vi "Instructor Log.vi"() -> ()   [LabVIEW 2017]
uses:
  <vilib>/OPCUA/controls/Write Status.ctl
  <vilib>/OPCUA/controls/NodeId.ctl
  <vilib>/OPCUA/client/Multiple Write String.vi
  <vilib>/OPCUA/NI OPC UA Client.lvlib
panel:
  out "Log Loop":i32
  out "Send Loop":i32
  in  "Stop Log":bool
  out "Chat Window":string
  in  "Node Status":T1 items=["Good"=0, "Uncertain_InitialValue"=1083310080, "Uncertain_LastUsableValue"=1083179008, "Uncertain_SensorNotAccurate"=1083375616, "Uncertain_EngineeringUnitsExceeded"=1083441152, "Bad_NoCommunication"=2150694912, "Bad_NotReadable"=2151284736, "Bad_NotWritable"=2151350272, "Bad_OutOfRange"=2151415808, "Bad_WaitingForInitialData"=2150760448]
  in  "Time Stamp":timestamp
  in  "Enter Text":string
  in  "Node Status":T1 items=["Good"=0, "Uncertain_InitialValue"=1083310080, "Uncertain_LastUsableValue"=1083179008, "Uncertain_SensorNotAccurate"=1083375616, "Uncertain_EngineeringUnitsExceeded"=1083441152, "Bad_NoCommunication"=2150694912, "Bad_NotReadable"=2151284736, "Bad_NotWritable"=2151350272, "Bad_OutOfRange"=2151415808, "Bad_WaitingForInitialData"=2150760448]
  in  "Time Stamp":timestamp
  in  "Stop Chat":bool
  in  "Send":bool
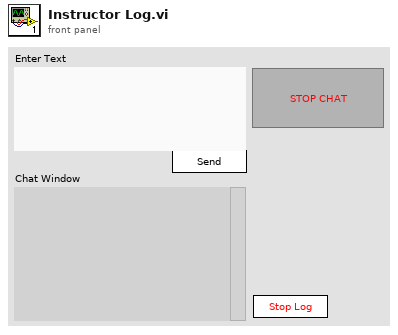
[diagram p1: front panel]
types:
  T1 = typedef "Write Status.ctl" = u32
  T2 = cluster{"message mode":enum16{"None", "Sign", "Sign and Encrypt"}, "security":enum16{"Basic256", "Basic128Rsa15"}}
  T3 = enum16{"open", "replace", "create", "open or create", "replace or create", "replace or create with confirmation"}
  T4 = typedef "OPC UA Client Refnum.ctl" = refnum<k21>
  T5 = typedef "NodeId.ctl" = string
  T6 = cluster{"node ID":T5, "value":string, "timestamp (current time)":timestamp, "node status":T1}
  T7 = cluster{"node ID":T5, "value":string, "timestamp (current time)":timestamp, "node status":T1}[]
  T8 = typedef "Subscription ID.ctl" = u32
  T9 = typedef "Subscription Data Change.ctl" = cluster{"node ID":T5, " value":variant, "timestamp":timestamp, "data type":T10, "status code":T11}
  T10 = typedef "Data Type.ctl" = u16
  T11 = typedef "OPC UA StatusCode.ctl" = u32
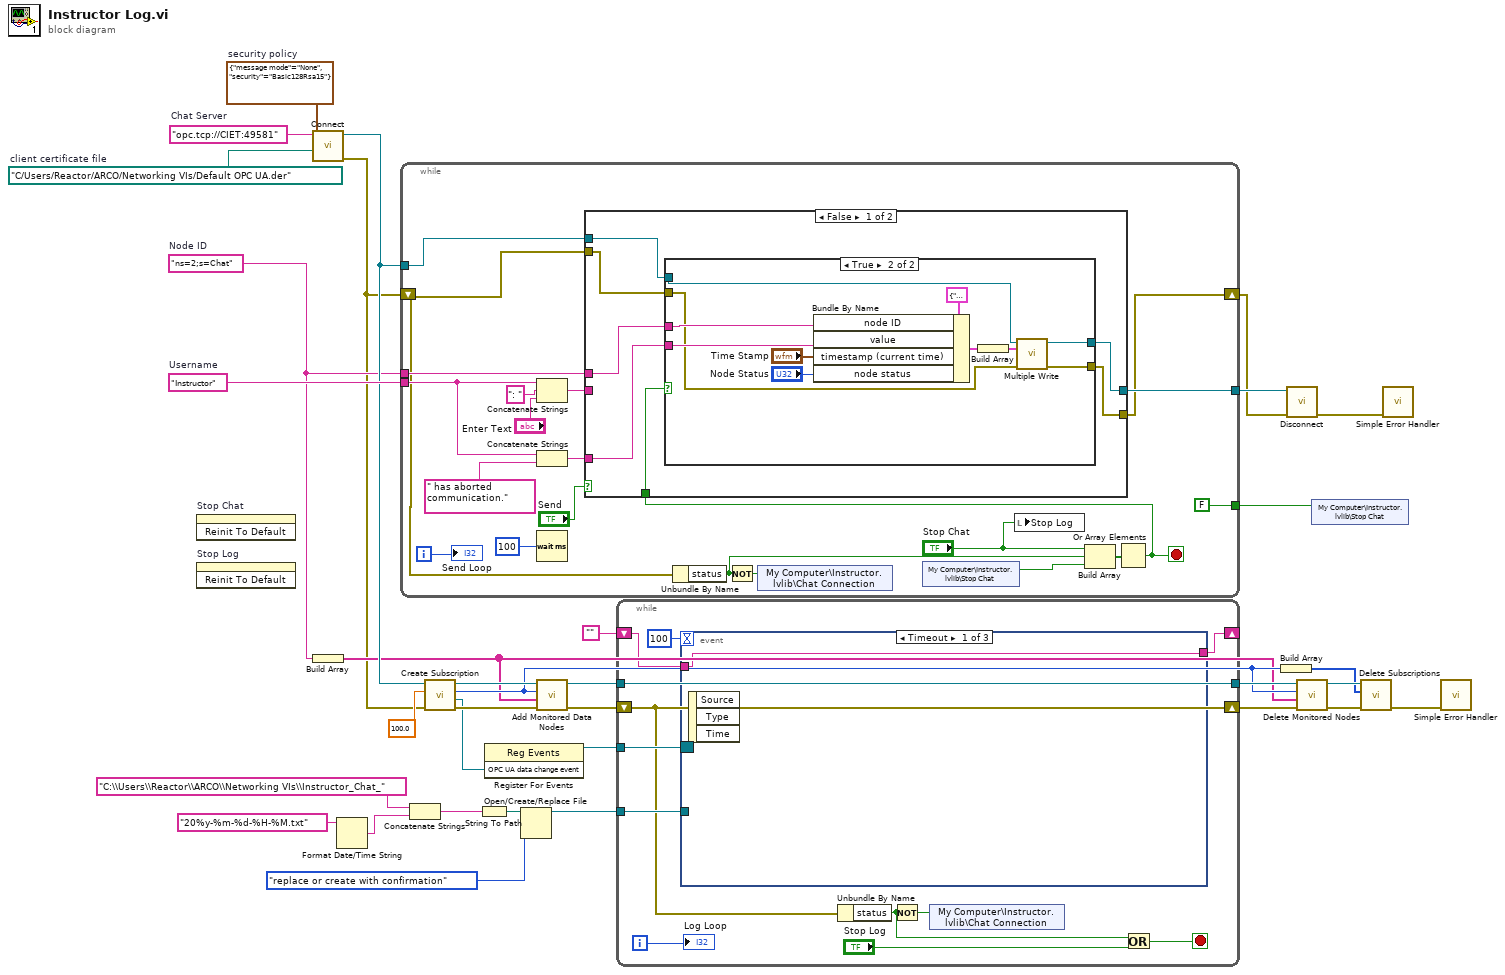
[diagram p0: block diagram]
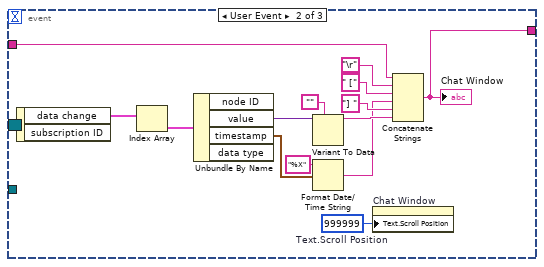
[diagram p2: hidden frame]
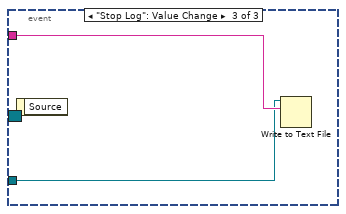
[diagram p3: hidden frame]
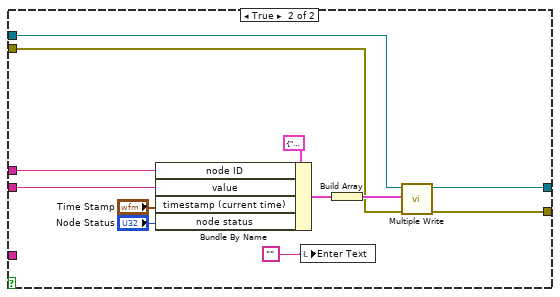
[diagram p5: hidden frame]
diagram:
  w12 = T2 {"message mode"=enum."None", "security"=enum."Basic128Rsa15"}  # security policy
  w13 = path "C:/Users/Reactor/ARCO/Networking VIs/Default OPC UA.der"  # client certificate file
  w17 = "ns=2;s=Chat"  # Node ID
  w32 = "Instructor"  # Username
  w33 = "opc.tcp://CIET:49581"  # Chat Server
  n1 = invoke on="Stop Chat" class="Bool (strict)" method="Reinit To Default"() -> ()  [unwired: 3 in, 3 out]
  n2 = invoke on="Stop Log" class="Bool (strict)" method="Reinit To Default"() -> ()  [unwired: 3 in, 3 out]
  n3 = call <vilib>:"Connect.vi"("client certificate file"=w13, "security policy"=w12, "server endpoint URL"=w33) -> ("error out"=w9:errorcluster, "OPC UA client refnum out"=w31:T4)  [unwired: 6 in, 1 out]
  n4 = Build Array(w17) -> (w16:string[])
  n5 = Format Date/Time String(time format string (%c)="20%y-%m-%d-%H-%M.txt") -> (date/time string=w4:string)  [unwired: 2 in]
  n6 = while {
    tunnel: w17 -> [w47]
    tunnel: w32 -> [w52]
    tunnel: w31 -> [w45]
    tunnel: [w46] -> w14
    tunnel: [FALSE] -> w10
    shift-right: [w36] -> w7
    shift-left: w9 -> [w35]
    i -> [w50]
    stop <- w41 stop-if-true
    n7 = Concatenate Strings(w52, ": ", "Enter Text") -> (w48:string)
    n8 = Concatenate Strings(w52, " has aborted communication.") -> (w44:string)
    n9 = Wait (ms)(milliseconds to wait=u32 100) -> ()  [unwired: 1 out]
    n10 = Unbundle By Name(w35) -> ("status"=w39:bool)
    n11 = Not(x=w39) -> (.not. x?=w42:bool)
    n12 = shared-variable "My Computer\\Instructor.lvlib\\Chat Connection"(w42) -> ()  [unwired: 1 in, 1 out]
    n13 = shared-variable "My Computer\\Instructor.lvlib\\Stop Chat"() -> (w40:bool)  [unwired: 1 in, 1 out]
    n14 = local write "Stop Log"("Stop Chat") -> ()
    n15 = Build Array("Stop Chat", w39, w40) -> (w37:bool[])
    n16 = Or Array Elements(Boolean array=w37) -> (logical OR=w41:bool)
    n17 = case shown="False" "Send" {
      tunnel: w48 -> [_ w82]
      tunnel: w47 -> [w60 w81]
      tunnel: [w56 w79] -> w46
      tunnel: [w57 w78] -> w36
      tunnel: w45 -> [w58 w77]
      tunnel: w35 -> [w59 w76]
      tunnel: w41 -> [w62 _]
      tunnel: w44 -> [w61 _]
      frame False {
        n18 = case shown="True" w62 {
          tunnel: w61 -> [_ w70]
          tunnel: w60 -> [_ w69]
          tunnel: w59 -> [w63 w68]
          tunnel: w58 -> [w64 w67]
          tunnel: [w64 w66] -> w56
          tunnel: [w63 w65] -> w57
          frame False {
          }
          frame True {
            n19 = Bundle By Name(cluster=T6 {"node ID"="", "value"="", "timestamp (current time)"=timestamp(0 s since 1904-01-01), "node status"=0} ("request"), "node ID"=w69, "value"=w70, "timestamp (current time)"="Time Stamp", "node status"="Node Status") -> (w73:T6)
            n20 = Build Array(w73) -> (w72:T7)
            n21 = call-poly <vilib>:"Multiple Write.vi"("error in (no error)"=w68, "requests"=w72, "OPC UA client refnum in"=w67) -> ("error out"=w65:errorcluster, "OPC UA client refnum out"=w66:T4)  [unwired: 5 in, 2 out]
          }
        }
      }
      frame True {
        n22 = Bundle By Name(cluster=T6 {"node ID"="", "value"="", "timestamp (current time)"=timestamp(0 s since 1904-01-01), "node status"=0} ("request"), "node ID"=w81, "value"=w82, "timestamp (current time)"="Time Stamp", "node status"="Node Status") -> (w85:T6)
        n23 = local write "Enter Text"("") -> ()
        n24 = Build Array(w85) -> (w84:T7)
        n25 = call-poly <vilib>:"Multiple Write.vi"("error in (no error)"=w76, "requests"=w84, "OPC UA client refnum in"=w77) -> ("error out"=w78:errorcluster, "OPC UA client refnum out"=w79:T4)  [unwired: 5 in, 2 out]
      }
    }
    "Send Loop" <- w50
  }
  n26 = Concatenate Strings("C:\\Users\\Reactor\\ARCO\\Networking VIs\\Instructor_Chat_" ("string"), w4) -> (w2:string)
  n27 = call <vilib>:"Create Subscription.vi"("error in (no error)"=w9, "publishing interval (1000 ms)"=100.0, "OPC UA client refnum in"=w31) -> ("error out"=w29:errorcluster, "OPC UA data change event"=w28:refnum<user-event>, "subscription ID out"=w21:T8, "OPC UA client refnum out"=w30:T4)  [unwired: 4 in, 1 out]
  n28 = String To Path(string=w2) -> (path=w3:path)
  n29 = register-events(w28) -> (reference out=w27:refnum<event-registration>)  [unwired: 2 in, 1 out]
  n30 = Open/Create/Replace File(file path (use dialog)=w3, operation (0:open)=T3."replace or create with confirmation") -> (refnum out=w18:refnum<file>)  [unwired: 4 in, 2 out]
  n31 = call <vilib>:"Add Monitored Data Nodes.vi"("error in (no error)"=w29, "node IDs"=w16, "subscription ID in"=w21, "OPC UA client refnum in"=w30) -> ("error out"=w8:errorcluster, "OPC UA client refnum out"=w25:T4)  [unwired: 4 in, 2 out]
  n32 = while {
    tunnel: w27 -> [w99]
    shift-right: [w97] -> _
    shift-left: "" -> [w98]
    tunnel: w25 -> [w96]
    tunnel: [w96] -> w24
    tunnel: w18 -> [w95]
    shift-right: [w88] -> w6
    shift-left: w8 -> [w88]
    i -> [w94]
    stop <- w90 stop-if-true
    n33 = event shown="[0] Timeout" {
      selector: w99 -> [_ _ _]
      dyn-events: _ -> [_ _ _]
      timeout: 100 -> [_ _ _]
      tunnel: w98 -> [w100 w103 w116]
      tunnel: [w100 w102 _] -> w97
      tunnel: w95 -> [_ _ w115]
      event Timeout {
        n34 = event-data() -> ()  [unwired: 1 in, 3 out]
      }
      event User Event {
        w101 = u32 999999  # Text.Scroll Position
        n35 = event-data() -> ("data change"=w114:T9[])  [unwired: 1 in, 1 out]
        n36 = Index Array(array=w114) -> (element=w113:T9)  [unwired: 1 in]
        n37 = Unbundle By Name(w113) -> ("value"=w112:variant, "timestamp"=w110:timestamp)  [unwired: 2 out]
        n38 = Variant To Data(type="", Variant=w112) -> (data=w108:string)  [unwired: 1 in, 1 out]
        n39 = Format Date/Time String(time format string (%c)="%X", seconds (now)=w110) -> (date/time string=w106:string)  [unwired: 1 in]
        n40 = property on="Chat Window" class="Str"("Text.Scroll Position"=w101) -> ()  [unwired: 2 in, 2 out]
        n41 = Concatenate Strings(w103, "\r", " [", w106, "] ", w108) -> (w102:string)
        "Chat Window" <- w102
      }
      event "Stop Log": Value Change {
        n42 = event-data() -> ()  [unwired: 1 in, 1 out]
        n43 = Write to Text File(file (use dialog)=w115, text=w116) -> ()  [unwired: 2 in, 3 out]
      }
    }
    n44 = Unbundle By Name(w88) -> ("status"=w92:bool)
    n45 = Not(x=w92) -> (.not. x?=w89:bool)
    n46 = shared-variable "My Computer\\Instructor.lvlib\\Chat Connection"(w89) -> ()  [unwired: 1 in, 1 out]
    n47 = Or(x=w92, y="Stop Log") -> (x .or. y?=w90:bool)
    "Log Loop" <- w94
  }
  n48 = Build Array(w21) -> (w20:T8[])
  n49 = call <vilib>:"Disconnect.vi"("error in (no error)"=w7, "OPC UA client refnum in"=w14) -> ("error out"=w34:errorcluster)  [unwired: 9 in]
  n50 = call <vilib>:"Delete Monitored Nodes.vi"("error in (no error)"=w6, "node IDs"=w16, "subscription ID in"=w21, "OPC UA client refnum in"=w24) -> ("error out"=w22:errorcluster, "OPC UA client refnum out"=w23:T4)  [unwired: 3 in, 3 out]
  n51 = shared-variable "My Computer\\Instructor.lvlib\\Stop Chat"(w10) -> ()  [unwired: 1 in, 1 out]
  n52 = call <vilib>:"Delete Subscriptions.vi"("error in (no error)"=w22, "subscription IDs"=w20, "OPC UA client refnum in"=w23) -> ("error out"=w19:errorcluster)  [unwired: 6 in, 2 out]
  n53 = call <vilib>:"Simple Error Handler.vi"("error in (no error)"=w34) -> ()  [unwired: 4 in, 5 out]
  n54 = call <vilib>:"Simple Error Handler.vi"("error in (no error)"=w19) -> ()  [unwired: 4 in, 5 out]
